vi "libssh2_session_init.vi"(8 "error in (no error)":errorcluster) -> (0 "error out":errorcluster, 3 "session":T1)   [LabVIEW 2013, in "libssh2.lvlib"]
doc: "Initializes a <B>session</B> object."
uses:
  libssh2.lvlib
  Session Refnum.ctl
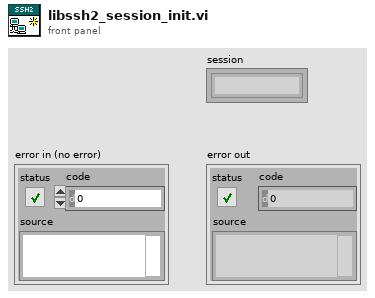
[diagram p1: front panel]
types:
  T1 = typedef "libssh2.lvlib/Session Refnum.ctl" = refnum<k1>
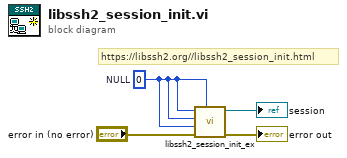
[diagram p0: block diagram]
diagram:
  w1 = u64 0  # NULL
  # "https://libssh2.org//libssh2_session_init.html"
  n1 = call "libssh2_session_init_ex.vi"("abstract"=w1, "error in (no error)"="error in (no error)", "myrealloc"=w1, "myfree"=w1, "myalloc"=w1) -> ("error out"=→"error out":errorcluster, "session"=→"session":T1)  [unwired: 5 in]
